vi "Cepilo_encerado.vi"() -> ()   [LabVIEW 2020]
panel:
  out "Cepillo encerado":bool
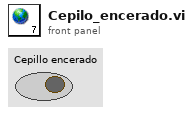
[diagram p1: front panel]
diagram:
